vi "ADIS16448 Loop Write Config.vi"(8 "error in (no error)":errorcluster, 11 "SPIDevRef":T1) -> (0 "error out":errorcluster, 3 "SPIDevRef out":T1)   [LabVIEW 2019]
uses:
  <vilib>/Rock Robotics/WPI/SPI/WPI_SPIDevRef.ctl
  <vilib>/Rock Robotics/SystemInterfaces/spilib/spi_bus.ctl
  Typedef/ADIS16448 Register.ctl
  <vilib>/Rock Robotics/WPI/SPI/WPI_SPIWrite.vi
  <vilib>/Utility/High Resolution Polling Wait.vi
  <vilib>/Rock Robotics/WPI/SPI/WPI_SPIRead.vi
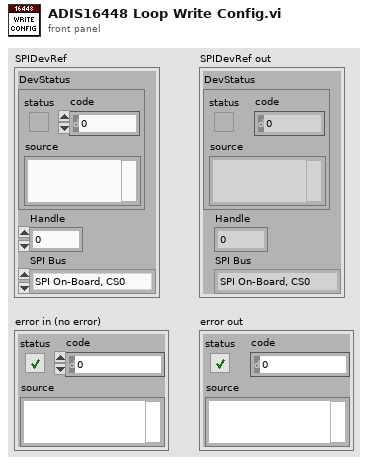
[diagram p1: front panel]
types:
  T1 = typedef "WPI_SPIDevRef.ctl" = cluster{"DevStatus":errorcluster, "Handle":i32, "SPI Bus":T2}
  T2 = typedef "spi_bus.ctl" = enum16{"SPI On-Board, CS0", "SPI On-Board, CS1", "SPI On-Board, CS2", "SPI On-Board, CS3", "SPI MXP", "Invalid"}
  T3 = typedef "ADIS16448 Register.ctl" = u8
  T4 = cluster{"Reg":T3, "Data":u16, "Write Config":bool}[]
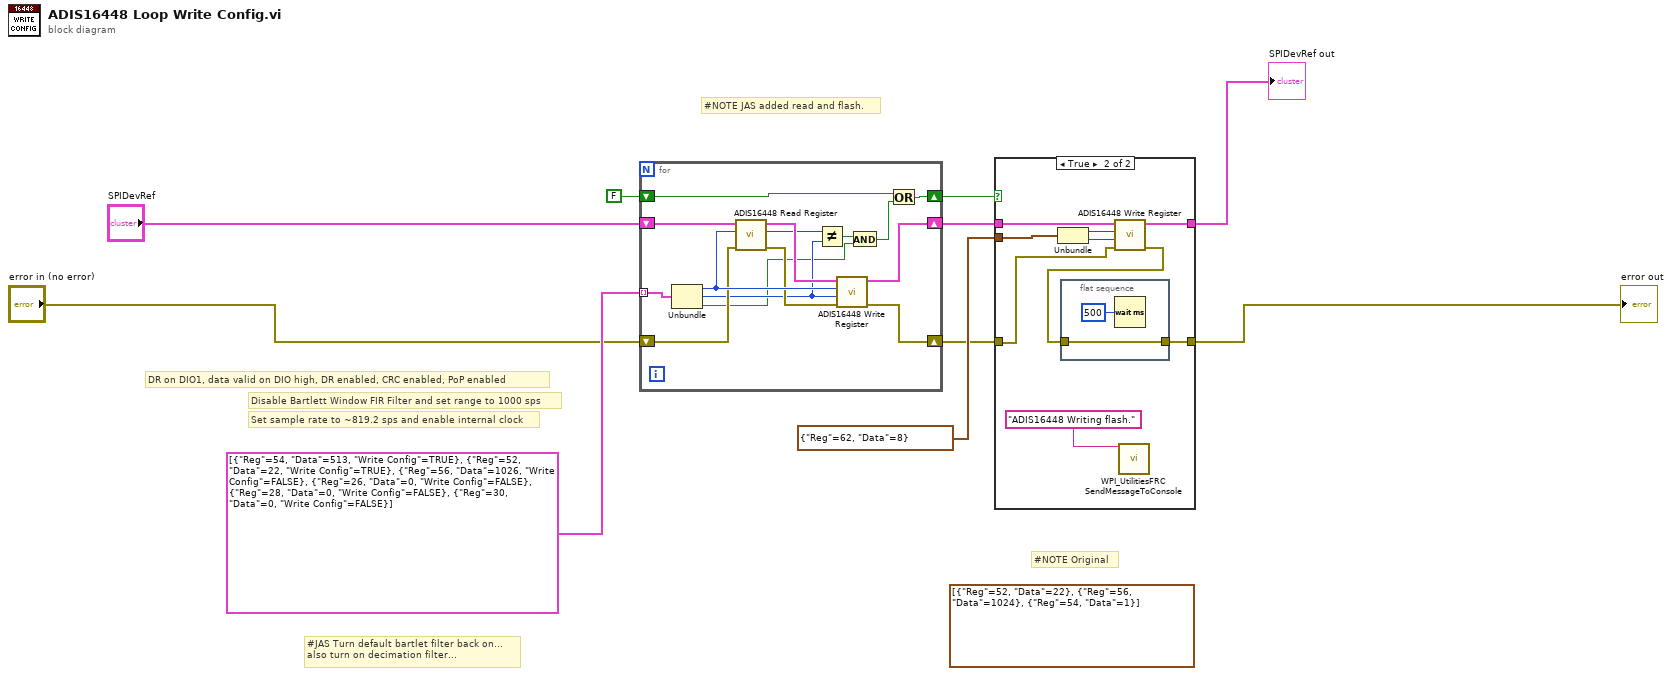
[diagram p0: block diagram]
diagram:
  (unwired) cluster{"Reg":T3, "Data":u16}[] [{"Reg"=52, "Data"=22}, {"Reg"=56, "Data"=1024}, {"Reg"=54, "Data"=1}]
  # "#JAS Turn default bartlet filter back on...\nalso turn on decimation filter..."
  # "#NOTE JAS added read and flash."
  # "#NOTE Original"
  # "DR on DIO1, data valid on DIO high, DR enabled, CRC enabled, PoP enabled"
  # "Set sample rate to ~819.2 sps and enable internal clock"
  # "Disable Bartlett Window FIR Filter and set range to 1000 sps"
  n1 = for {
    tunnel: T4 [{"Reg"=54, "Data"=513, "Write Config"=TRUE}, {"Reg"=52, "Data"=22, "Write Config"=TRUE}, {"Reg"=56, "Data"=1026, "Write Config"=FALSE}, {"Reg"=26, "Data"=0, "Write Config"=FALSE}, {"Reg"=28, "Data"=0, "Write Config"=FALSE}, {"Reg"=30, "Data"=0, "Write Config"=FALSE}] -> [w25] mode=indexing
    shift-right: [w24] -> w8
    shift-left: "error in (no error)" -> [w18]
    shift-right: [w23] -> w6
    shift-left: "SPIDevRef" -> [w22]
    shift-right: [w16] -> w5
    shift-left: FALSE -> [w17]
    n2 = Unbundle(w25) -> ("Reg"=w21:T3, "Data"=w14:u16, "Write Config"=w11:bool)
    n3 = call "ADIS16448 Read Register.vi"("error in (no error)"=w18, "ADIS16448 Register"=w21, "SPIDevRef in"=w22) -> ("error out"=w19:errorcluster, "Register Value"=w15:u16, "SPIDevRef out"=w20:T1)  [unwired: 6 in]
    n4 = Not Equal?(x=w15, y=w14) -> (x != y?=w13:bool)
    n5 = call "ADIS16448 Write Register.vi"("error in (no error)"=w19, "Data"=w14, "Register"=w21, "SPIDevRef in"=w20) -> ("error out"=w24:errorcluster, "SPIDevRef out"=w23:T1)  [unwired: 6 in]
    n6 = And(x=w13, y=w11) -> (x .and. y?=w12:bool)
    n7 = Or(x=w17, y=w12) -> (x .or. y?=w16:bool)
  }
  n8 = case shown="True" w5 {
    tunnel: w6 -> [w27 w35]
    tunnel: [w27 w36] -> w7
    tunnel: w8 -> [w26 w34]
    tunnel: [w26 w32] -> w9
    tunnel: cluster{"Reg":T3, "Data":i32} {"Reg"=62, "Data"=8} -> [_ w31]
    frame False {
    }
    frame True {
      n9 = Unbundle(w31) -> ("Reg"=w30:T3, "Data"=w29:i32)
      n10 = flat-sequence {
        tunnel: [w38] -> w32
        tunnel: w33 -> [w38]
        frame #0 {
          n11 = Wait (ms)(milliseconds to wait=u32 500) -> ()  [unwired: 1 out]
        }
      }
      n12 = call "ADIS16448 Write Register.vi"("error in (no error)"=w34, "Data"=w29, "Register"=w30, "SPIDevRef in"=w35) -> ("error out"=w33:errorcluster, "SPIDevRef out"=w36:T1)  [unwired: 6 in]
      n13 = call <vilib>:"WPI_UtilitiesFRC SendMessageToConsole.vi"("Message"="ADIS16448 Writing flash." ("format string")) -> ()  [unwired: 14 in, 1 out]
    }
  }
  "error out" <- w9
  "SPIDevRef out" <- w7
